vi "Logger.File.PropertiesRead.vi"(8 "error in (no error)":errorcluster, 11 "file path":path) -> (0 "error out":errorcluster, 2 "Properties":T1, 3 "File ref out":refnum<k34>, 5 "Ref":string)   [LabVIEW 2016]
uses:
  Logger.File.Properties.ctl
  Sequence/Sequence.Code.SerialFormat.ctl
  Sequence/Sequence.Counters.ctl
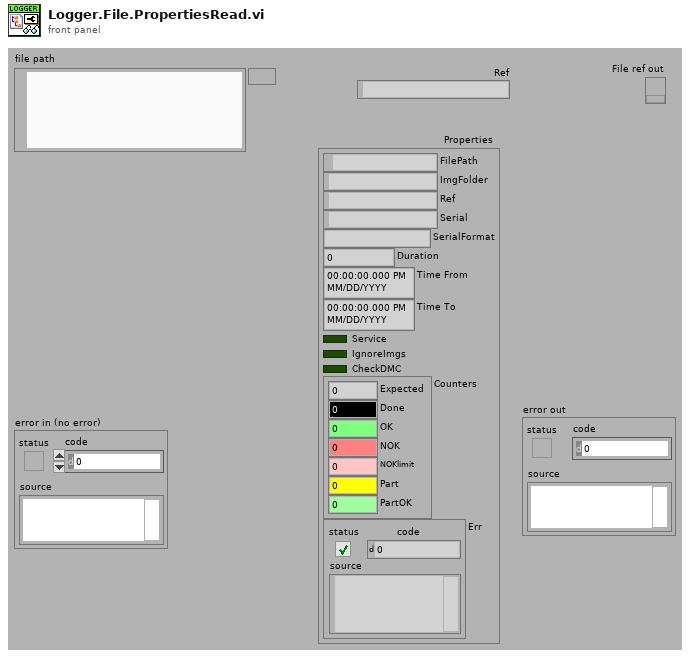
[diagram p1: front panel]
types:
  T1 = typedef "Logger.File.Properties.ctl" = cluster{"FilePath":path, "ImgFolder":string, "Ref":string, "Serial":string, "SerialFormat":T2, "Duration":dbl, "Time From":timestamp, "Time To":timestamp, "Service":bool, "IgnoreImgs":bool, "CheckDMC":bool, "Counters":T3, "Err":errorcluster}
  T2 = typedef "Sequence.Code.SerialFormat.ctl" = enum8{"", "6 dig", "7 dig"}
  T3 = typedef "Sequence.Counters.ctl" = cluster{"Expected":u16, "Done":u16, "OK":u16, "NOK":u16, "NOKlimit":u16, "Part":u16, "PartOK":u16}
  T4 = enum16{"open", "open or create", "create or replace", "create", "open (read-only)"}
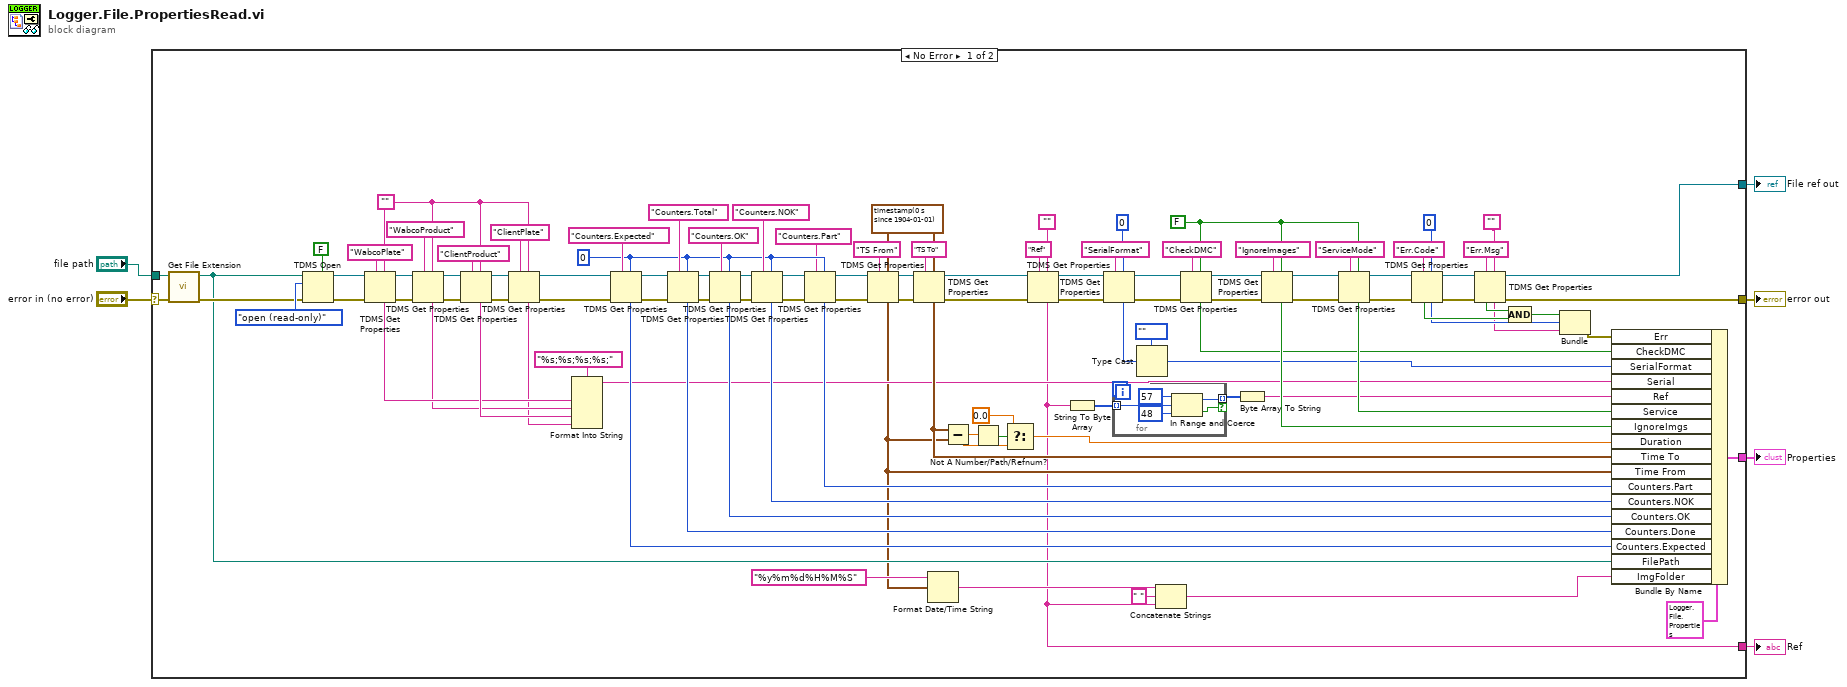
[diagram p0: block diagram]
diagram:
  n1 = case shown="No Error" "error in (no error)" {
    selector: "error in (no error)" -> [w101 w121]
    tunnel: [w88 w121] -> w4
    tunnel: "file path" -> [w102 _]
    tunnel: [w99 _] -> w3
    tunnel: [w86 _] -> w2
    tunnel: [w7 _] -> w1
    frame No Error {
      w50 = ""
      w21 = FALSE
      w40 = u16 0
      w109 = timestamp(0 s since 1904-01-01)
      n2 = call <vilib>:"Get File Extension.vi"("error in (no error)"=w101, "file"=w102) -> ("error out"=w100:errorcluster, "dup file"=w97:path)  [unwired: 5 in, 3 out]
      n3 = TDMS Open(5:FALSE ("create index file? (T)"), 8:w100, 10:T4."open (read-only)" ("operation (0:open)"), 11:w97) -> (0:w48:errorcluster, 3:w45:refnum<k34>)  [unwired: 3 in]
      n4 = TDMS Get Properties(5:w50, 7:"WabcoPlate", 8:w48, 11:w45) -> (0:w59:errorcluster, 3:w60:refnum<k34>, 4:w26:string)  [unwired: 2 in, 3 out]
      n5 = TDMS Get Properties(5:w50, 7:"WabcoProduct", 8:w59, 11:w60) -> (0:w55:errorcluster, 3:w56:refnum<k34>, 4:w25:string)  [unwired: 2 in, 3 out]
      n6 = TDMS Get Properties(5:w50, 7:"ClientProduct", 8:w55, 11:w56) -> (0:w58:errorcluster, 3:w57:refnum<k34>, 4:w49:string)  [unwired: 2 in, 3 out]
      n7 = TDMS Get Properties(5:w50, 7:"ClientPlate", 8:w58, 11:w57) -> (0:w47:errorcluster, 3:w46:refnum<k34>, 4:w24:string)  [unwired: 2 in, 3 out]
      n8 = Format Into String(format string="%s;%s;%s;%s;", w26, w25, w49, w24) -> (resulting string=w23:string)  [unwired: 2 in, 1 out]
      n9 = TDMS Get Properties(5:w40, 7:"Counters.Expected" ("property name"), 8:w47, 11:w46) -> (0:w72:errorcluster, 3:w73:refnum<k34>, 4:w70:u16)  [unwired: 2 in, 3 out]
      n10 = TDMS Get Properties(5:w40, 7:"Counters.Total", 8:w72, 11:w73) -> (0:w64:errorcluster, 3:w63:refnum<k34>, 4:w69:u16)  [unwired: 2 in, 3 out]
      n11 = TDMS Get Properties(5:w40, 7:"Counters.OK" ("property name"), 8:w64, 11:w63) -> (0:w67:errorcluster, 3:w66:refnum<k34>, 4:w61:u16)  [unwired: 2 in, 3 out]
      n12 = TDMS Get Properties(5:w40, 7:"Counters.NOK", 8:w67, 11:w66) -> (0:w38:errorcluster, 3:w39:refnum<k34>, 4:w62:u16)  [unwired: 2 in, 3 out]
      n13 = TDMS Get Properties(5:w40, 7:"Counters.Part", 8:w38, 11:w39) -> (0:w37:errorcluster, 3:w36:refnum<k34>, 4:w34:u16)  [unwired: 2 in, 3 out]
      n14 = TDMS Get Properties(5:w109, 7:"TS From" ("property name"), 8:w37, 11:w36) -> (0:w112:errorcluster, 3:w111:refnum<k34>, 4:w13:timestamp)  [unwired: 2 in, 3 out]
      n15 = TDMS Get Properties(5:w109, 7:"TS To" ("property name"), 8:w112, 11:w111) -> (0:w76:errorcluster, 3:w75:refnum<k34>, 4:w96:timestamp)  [unwired: 2 in, 3 out]
      n16 = Format Date/Time String(time format string (%c)="%y%m%d%H%M%S", seconds (now)=w13) -> (date/time string=w9:string)  [unwired: 1 in]
      n17 = Subtract(x=w96, y=w13) -> (x-y=w79:dbl)
      n18 = Not A Number/Path/Refnum?(number/path/refnum=w79) -> (NaN/Path/Refnum?=w80:bool)
      n19 = Select(t=0.0, s=w80, f=w79) -> (s? t:f=w11:dbl)
      n20 = TDMS Get Properties(5:"", 7:"Ref" ("property name"), 8:w76, 11:w75) -> (0:w30:errorcluster, 3:w31:refnum<k34>, 4:w7:string)  [unwired: 2 in, 3 out]
      n21 = String To Byte Array(string=w7) -> (unsigned byte array=w43:u8[])
      n22 = TDMS Get Properties(5:u8 0, 7:"SerialFormat" ("property name"), 8:w30, 11:w31) -> (0:w16:errorcluster, 3:w19:refnum<k34>, 4:w29:u8)  [unwired: 2 in, 3 out]
      n23 = for {
        tunnel: w43 -> [w120] mode=indexing
        tunnel: [w117] -> w42 mode=indexing if=w116
        n24 = In Range and Coerce(upper limit=u8 57, x=w120, lower limit=u8 48) -> (coerced(x)=w117:u8, In Range?=w116:bool)
      }
      n25 = Type Cast(type=Sequence.Code.SerialFormat."" ("SerialFormat"), x=w29) -> (*(type *) &x=w27:T2)
      n26 = Concatenate Strings(w9, " " ("string"), w7) -> (w10:string)
      n27 = TDMS Get Properties(5:w21, 7:"CheckDMC" ("property name"), 8:w16, 11:w19) -> (0:w17:errorcluster, 3:w18:refnum<k34>, 4:w15:bool)  [unwired: 2 in, 3 out]
      n28 = Byte Array To String(unsigned byte array=w42) -> (string=w41:string)
      n29 = TDMS Get Properties(5:w21, 7:"IgnoreImages" ("property name"), 8:w17, 11:w18) -> (0:w105:errorcluster, 3:w104:refnum<k34>, 4:w74:bool)  [unwired: 2 in, 3 out]
      n30 = TDMS Get Properties(5:w21, 7:"ServiceMode" ("property name"), 8:w105, 11:w104) -> (0:w90:errorcluster, 3:w87:refnum<k34>, 4:w103:bool)  [unwired: 2 in, 3 out]
      n31 = TDMS Get Properties(5:0, 7:"Err.Code" ("property name"), 8:w90, 11:w87) -> (0:w89:errorcluster, 3:w95:refnum<k34>, 4:w83:i32, 6:w84:bool)  [unwired: 2 in, 2 out]
      n32 = TDMS Get Properties(5:"", 7:"Err.Msg" ("property name"), 8:w89, 11:w95) -> (0:w88:errorcluster, 3:w86:refnum<k34>, 4:w82:string, 6:w85:bool)  [unwired: 2 in, 2 out]
      n33 = Compound Arithmetic op=AND(w85, w84) -> (w81:bool)
      n34 = Bundle(w81, w83, w82) -> (w12:errorcluster)  [unwired: 1 in]
      n35 = Bundle By Name(cluster=T1 {"FilePath"=path "", "ImgFolder"="", "Ref"="", "Serial"="", "SerialFormat"=enum."", "Duration"=0.0, "Time From"=timestamp(0 s since 1904-01-01), "Time To"=timestamp(0 s since 1904-01-01), "Service"=FALSE, "IgnoreImgs"=FALSE, "CheckDMC"=FALSE, "Counters"={"Expected"=0, "Done"=0, "OK"=0, "NOK"=0, "NOKlimit"=0, "Part"=0, "PartOK"=0}, "Err"={"status"=FALSE, "code"=0, "source"=""}} ("Properties"), "Err"=w12, "CheckDMC"=w15, "SerialFormat"=w27, "Serial"=w23, "Ref"=w41, "Service"=w103, "IgnoreImgs"=w74, "Duration"=w11, "Time To"=w96, "Time From"=w13, "Counters.Part"=w34, "Counters.NOK"=w62, "Counters.OK"=w61, "Counters.Done"=w69, "Counters.Expected"=w70, "FilePath"=w97, "ImgFolder"=w10) -> (w99:T1)
    }
    frame Error {
    }
  }
  "error out" <- w4
  "Properties" <- w3
  "File ref out" <- w2
  "Ref" <- w1
